vi "AnyBuilderBuild.vi"(8 "error in":errorcluster, 10 "Message Type":string, 11 "Builder Ref":T2) -> (0 "error out":errorcluster, 3 "Any":T1)   [LabVIEW 2019, in "grpc-lvsupport.lvlib"]
uses:
  grpc-lvsupport.lvlib
  Shared/grpcId.ctl
  Shared/Any.ctl
  <vilib>/AdvancedString/1D String Array to Delimited String.vi
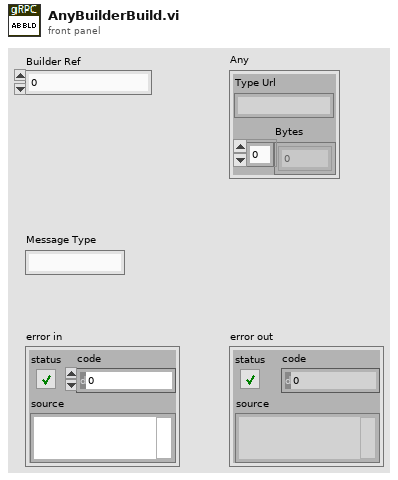
[diagram p1: front panel]
types:
  T1 = typedef "grpc-lvsupport.lvlib/Any.ctl" = cluster{"Type Url":string, "Bytes":u8[]}
  T2 = typedef "grpc-lvsupport.lvlib/grpcId.ctl" = u64
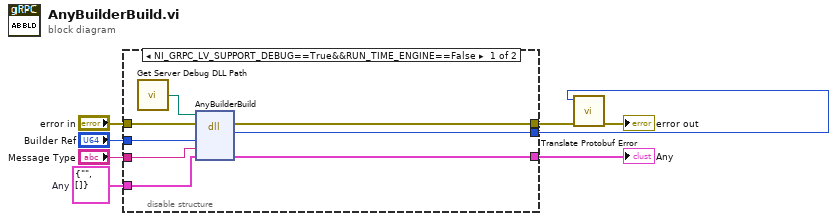
[diagram p0: block diagram]
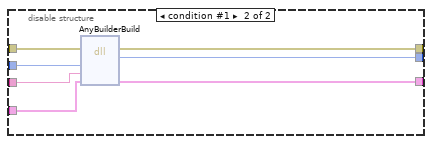
[diagram p2: hidden frame]
diagram:
  w4 = T1 {"Type Url"="", "Bytes"=[]}  # Any
  n1 = disable-structure shown="NI_GRPC_LV_SUPPORT_DEBUG==True&&RUN_TIME_ENGINE==False" {
    disable-tunnel: "error in" -> [w16 w23]
    disable-tunnel: [w15 w22] -> w7
    disable-tunnel: "Builder Ref" -> [w13 w21]
    disable-tunnel: "Message Type" -> [w12 w20]
    disable-tunnel: w4 -> [w11 w19]
    disable-tunnel: [w10 w18] -> w3
    disable-tunnel: [w9 w17] -> w1
    frame condition #0 (active) {
      n2 = call "Get Server Debug DLL Path.vi"() -> ("Server Debug DLL Path"=w14:path)
      n3 = dll-call lib="?" fn="AnyBuilderBuild"(path in=w14, error in=w16, "builderId"=w13, "messageType"=w12, "any"=w11) -> (error out=w15:errorcluster, "return type"=w9:i32, "any"=w10:T1)  [unwired: 3 in, 1 out]
    }
    frame condition #1 {
      n4 = dll-call lib="?" fn="AnyBuilderBuild"(error in=w23, "builderId"=w21, "messageType"=w20, "any"=w19) -> (error out=w22:errorcluster, "return type"=w17:i32, "any"=w18:T1)  [unwired: 4 in, 1 out]
    }
  }
  "Any" <- w3
  n5 = call "Translate Protobuf Error.vi"("error in"=w7, "Error Code"=w1) -> ("error out"=→"error out":errorcluster)  [unwired: 9 in]
